vi "ECG_WD.vi"() -> ()   [LabVIEW 2020]
uses:
  <vilib>/Analysis/3filter.llb/Filter Passband Type.ctl
  <vilib>/Analysis/2dsp.llb/Real FFT.vi
  <vilib>/Utility/file.llb/Read Delimited Spreadsheet (DBL).vi
  <vilib>/Analysis/3filter.llb/Butterworth Filter (DBL).vi
  <vilib>/Analysis/NI_AALBase.lvlib
  <vilib>/Analysis/NI_AALPro.lvlib
panel:
  out "WD_stimuli 4":dbl[](graph)
  out "WD_stimuli3":dbl[](graph)
  out "WD_stimuli 2":dbl[](graph)
  out "WD_stimuli1":dbl[](graph)
  out "WD_baseline":dbl[](graph)
  out "PS_WD_stimuli4":cluster{"x":dbl, "x":dbl, dbl[]}(graph)
  out "PS_WD_stimuli 2":cluster{"x":dbl, "x":dbl, dbl[]}(graph)
  out "PS_WD_stimuli3":cluster{"x":dbl, "x":dbl, dbl[]}(graph)
  out "PS_WD_stimuli1":cluster{"x":dbl, "x":dbl, dbl[]}(graph)
  out "PS_WD_baseline 2":cluster{"x":dbl, "x":dbl, dbl[]}(graph)
  out "RRI_series_WD_stimuli4":dbl[](graph)
  out "RRI_series_WD_stimuli3":dbl[](graph)
  out "RRI_series_WD_stimuli2":dbl[](graph)
  out "RRI_series_WD_stimuli1":dbl[](graph)
  out "RRI_series_WD_baseline":dbl[](graph)
  out "WD_stimuli 4":dbl[](graph)
  out "WD_stimuli3":dbl[](graph)
  out "WD_stimuli 2":dbl[](graph)
  out "WD_stimuli1":dbl[](graph)
  out "WD_baseline":dbl[](graph)
  out "psd_size 5":i32
  out "PS_WD_stimuli4":cluster{"x":dbl, "x":dbl, dbl[]}(graph)
  out "LF/HF 5":dbl
  out "HF  2":dbl
  out "LF  2":dbl
  out "TP (<=0.4Hz)  2":dbl
  out "RRI_size 5":i32
  out "RRI_series_WD_stimuli4":dbl[](graph)
  out "RRI series 5":dbl[](array[numeric])
  out "size(s) 5":i32
  out "2nd Derivatives 5":dbl[](array[numeric])
  out "Amplitudes 5":dbl[](array[numeric])
  out "amplitude 5":dbl[](array[numeric])
  out "location 5":dbl[](array[numeric])
  out "Locations 5":dbl[](array[numeric])
  in  "file path (dialog if empty) 5":path
  out "psd_size 4":i32
  out "PS_WD_stimuli3":cluster{"x":dbl, "x":dbl, dbl[]}(graph)
  out "LF/HF 4":dbl
  out "HF  2":dbl
  out "LF  2":dbl
  out "TP (<=0.4Hz)  2":dbl
  out "RRI_size 4":i32
  out "RRI_series_WD_stimuli3":dbl[](graph)
  out "RRI series 4":dbl[](array[numeric])
  out "size(s) 4":i32
  out "2nd Derivatives 4":dbl[](array[numeric])
  out "Amplitudes 4":dbl[](array[numeric])
  out "amplitude 4":dbl[](array[numeric])
  out "location 4":dbl[](array[numeric])
  out "Locations 4":dbl[](array[numeric])
  in  "file path (dialog if empty) 4":path
  out "psd_size 3":i32
  out "PS_WD_stimuli 2":cluster{"x":dbl, "x":dbl, dbl[]}(graph)
  out "LF/HF 3":dbl
  out "HF  2":dbl
  out "LF  2":dbl
  out "TP (<=0.4Hz)  2":dbl
  out "RRI_size 3":i32
  out "RRI_series_WD_stimuli2":dbl[](graph)
  out "RRI series 3":dbl[](array[numeric])
  out "size(s) 3":i32
  out "2nd Derivatives 3":dbl[](array[numeric])
  out "Amplitudes 3":dbl[](array[numeric])
  out "amplitude 3":dbl[](array[numeric])
  out "location 3":dbl[](array[numeric])
  out "Locations 3":dbl[](array[numeric])
  in  "file path (dialog if empty) 3":path
  out "psd_size 2":i32
  out "PS_WD_stimuli1":cluster{"x":dbl, "x":dbl, dbl[]}(graph)
  out "LF/HF 2":dbl
  out "HF  2":dbl
  out "LF  2":dbl
  out "TP (<=0.4Hz)  2":dbl
  out "RRI_size 2":i32
  out "RRI_series_WD_stimuli1":dbl[](graph)
  out "RRI series 2":dbl[](array[numeric])
  out "size(s) 2":i32
  out "2nd Derivatives 2":dbl[](array[numeric])
  out "Amplitudes 2":dbl[](array[numeric])
  out "amplitude 2":dbl[](array[numeric])
  out "location 2":dbl[](array[numeric])
  out "Locations 2":dbl[](array[numeric])
  in  "file path (dialog if empty) 2":path
  out "psd_size":i32
  out "PS_WD_baseline":cluster{"x":dbl, "x":dbl, dbl[]}(graph)
  out "LF/HF":dbl
  out "HF":dbl
  out "LF":dbl
  out "TP (<=0.4Hz)":dbl
  out "RRI_size":i32
  out "RRI_series_WD_baseline":dbl[](graph)
  out "RRI series":dbl[](array[numeric])
  out "size(s)":i32
  out "2nd Derivatives":dbl[](array[numeric])
  out "Amplitudes":dbl[](array[numeric])
  out "amplitude":dbl[](array[numeric])
  out "location":dbl[](array[numeric])
  out "Locations":dbl[](array[numeric])
  in  "file path (dialog if empty)":path
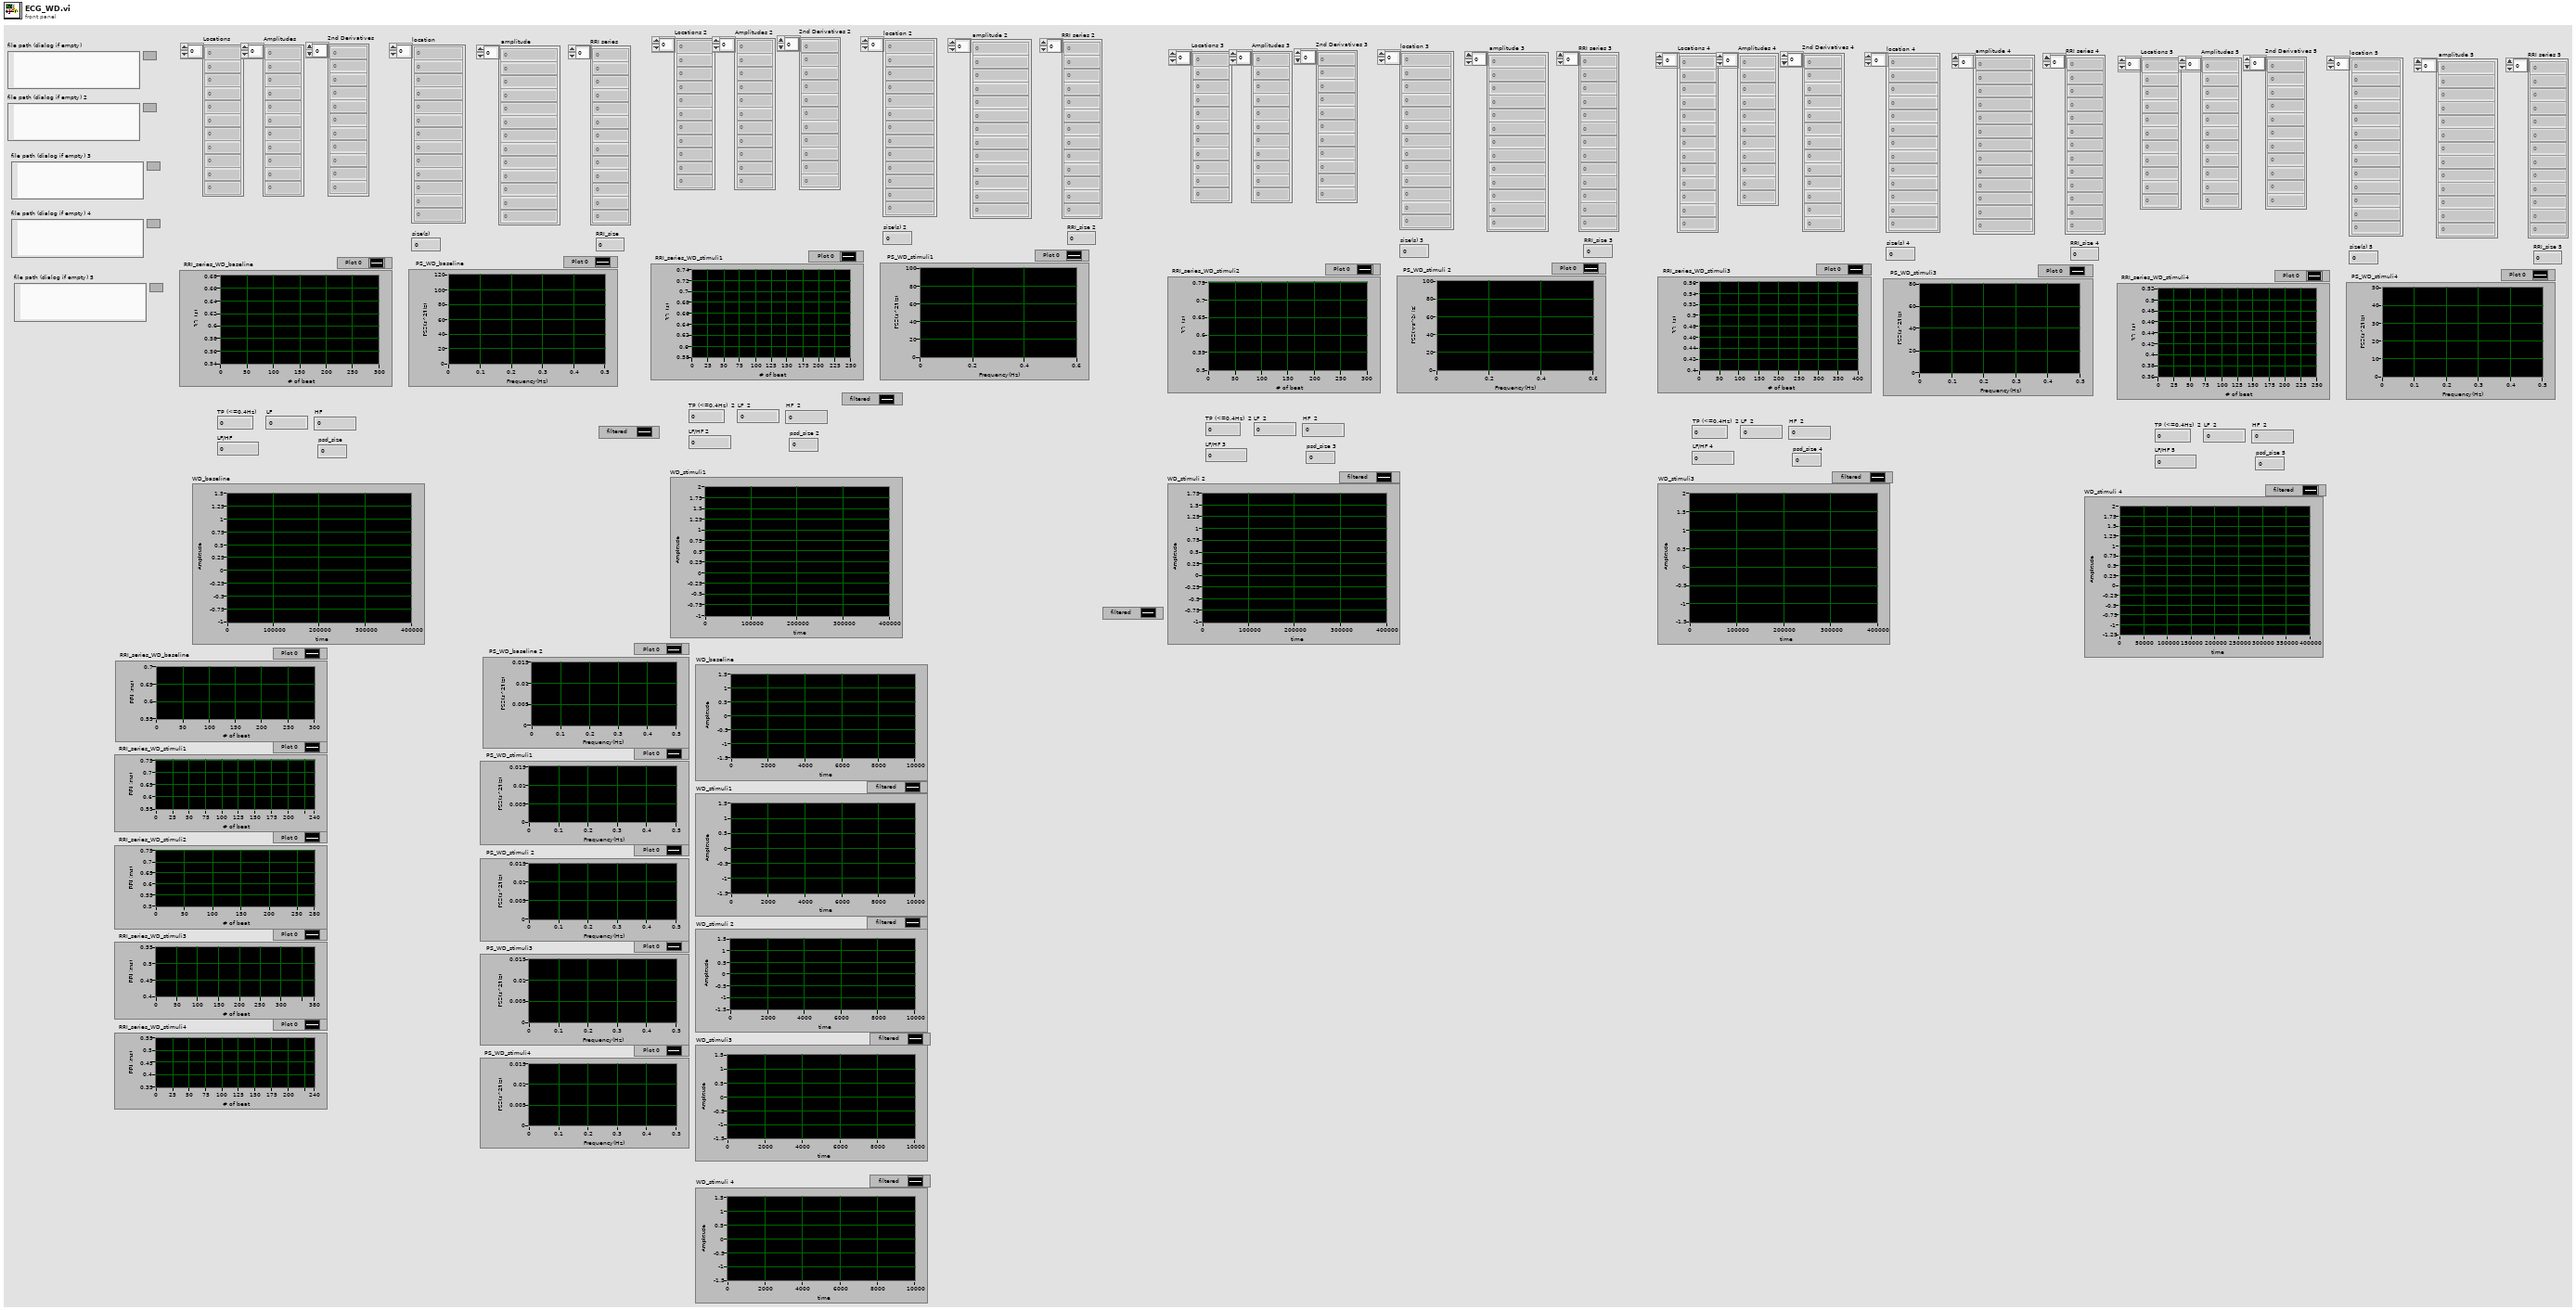
[diagram p1: front panel]
types:
  T1 = typedef "NI_AALBase.lvlib/Filter Passband Type.ctl" = enum32{"Lowpass", "Highpass", "Bandpass", "Bandstop"}
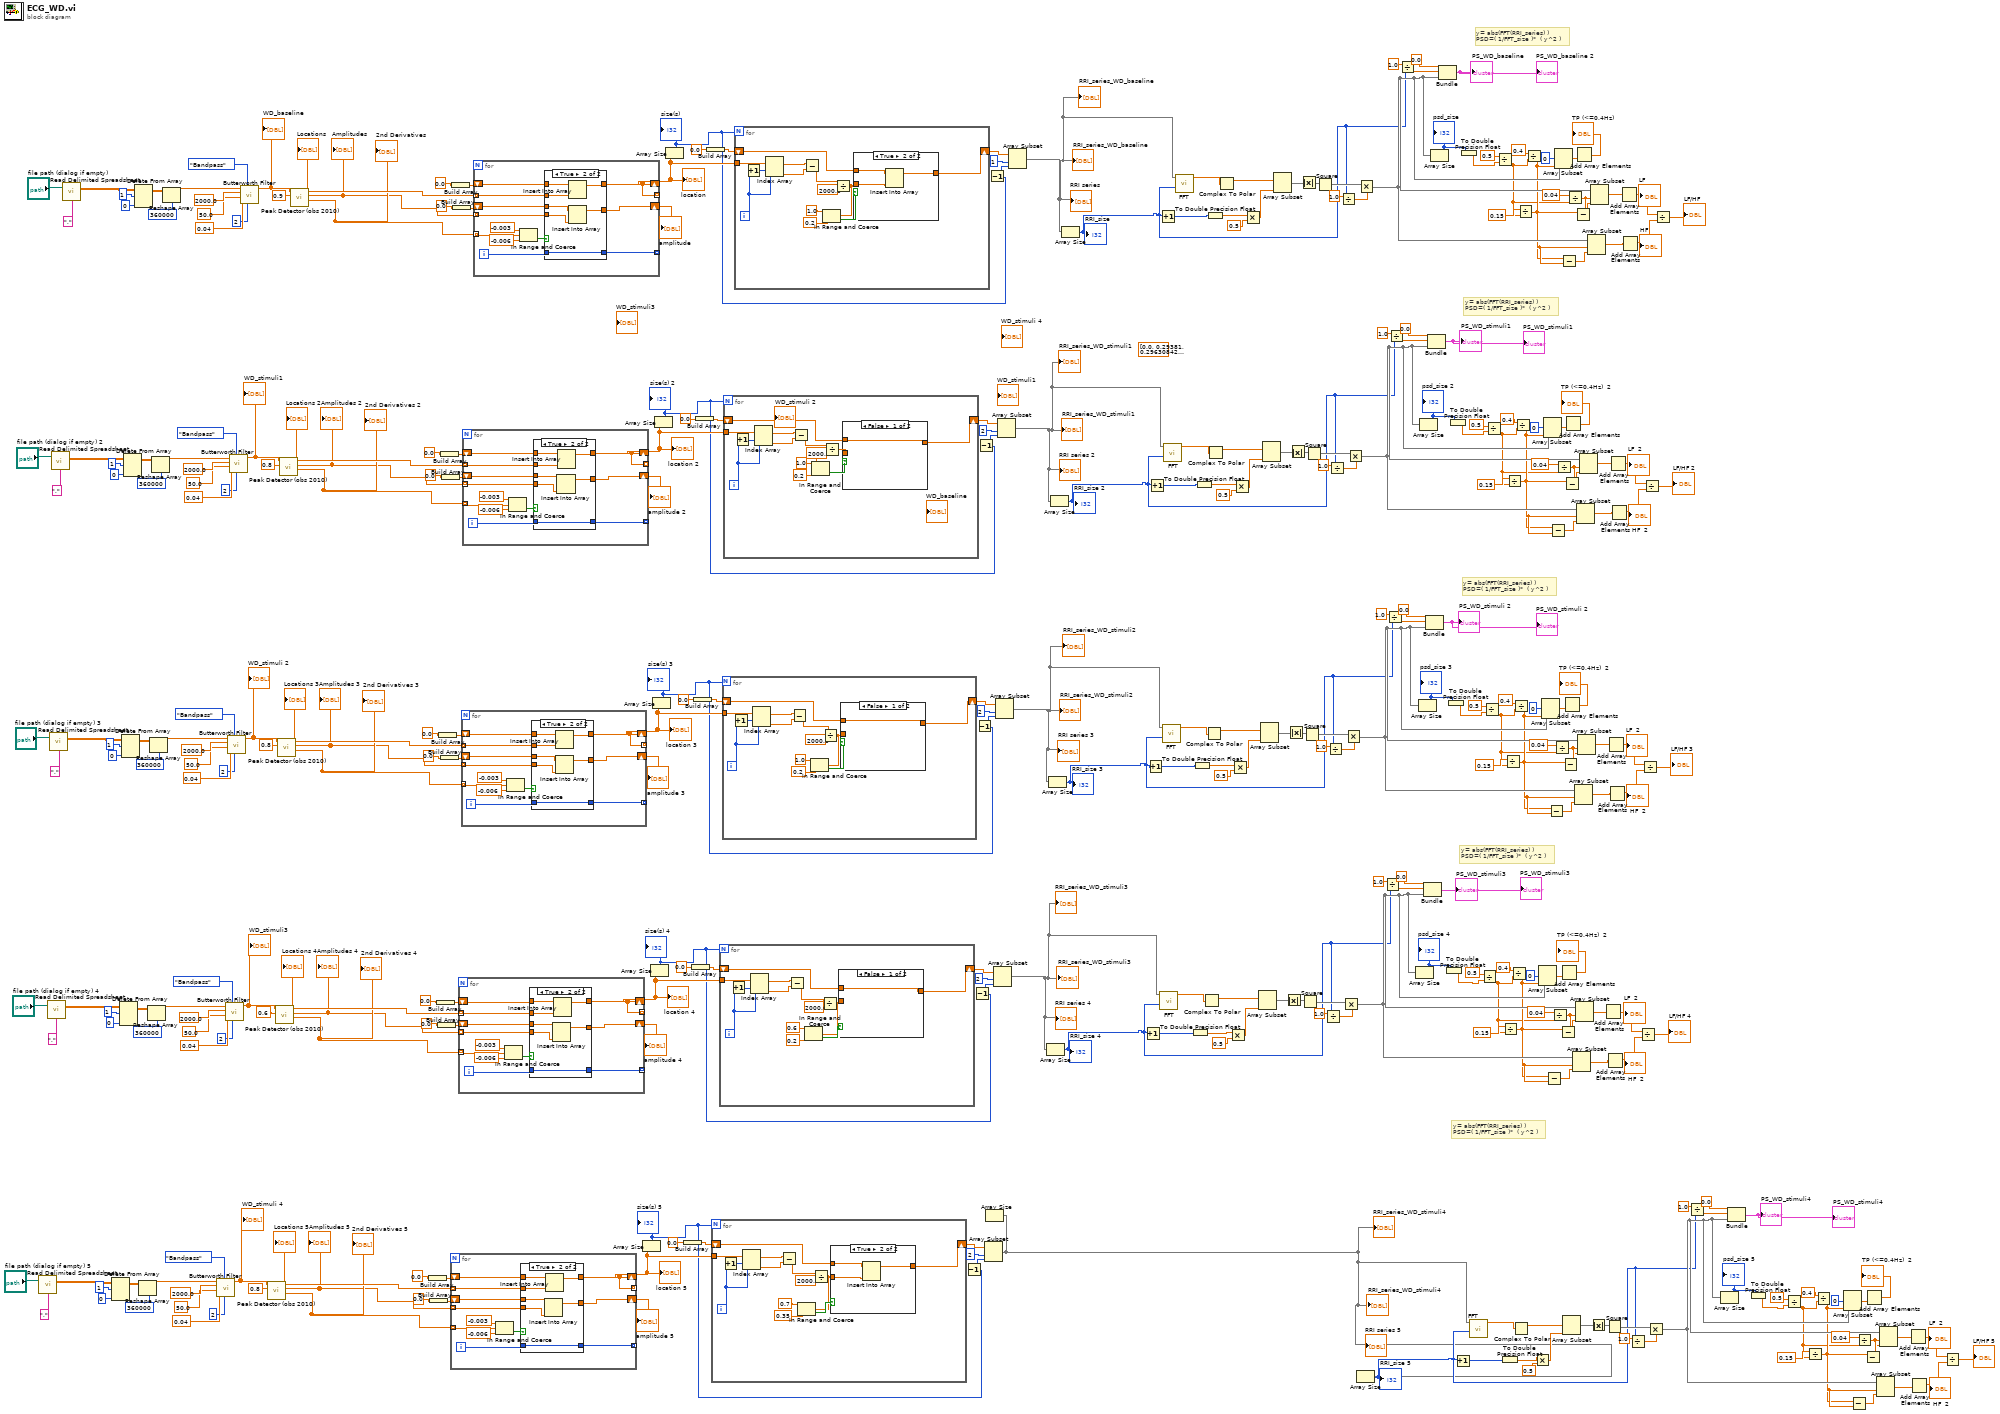
[diagram p0: block diagram]
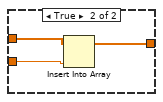
[diagram p4: hidden frame]
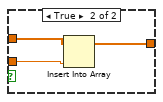
[diagram p6: hidden frame]
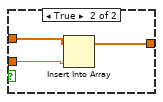
[diagram p8: hidden frame]
diagram:
  (unwired) dbl[] [0.0, 0.29381, 0.29630842105263167, 0.19107985480943712, 0.38411172413793127, 0.2005576470588235, 0.5415192546583851, 0.45620357142857126, 0.38751630434782625, 0.5665753623188401, 0.15213750000000026, 0.5900847665847664, 0.5553697788697791, 0.2967545454545455, 0.25331290322580635, 0.24809710144927521, 0.24300555555555636, 0.36543567251461884, 0.21673793859649226, 0.5703541666666663, 0.5683518808777421, 0.1222697768762675, 0.18815601023018047, 0.5246007905138335, 0.1950573913043474, 0.33014545454545363, 0.44885793103448357, 0.23535953177257518, 0.22516909814323682, 0.22548551724137944, 0.12783937499999887, 0.3413281250000004, 0.20749715909090938, 0.4030790441176464, 0.23350756302520992, 0.21006071428571715, 0.11335771889400803, 0.22295537634408547, 0.26558703703703657, 0.539833333333334, 0.10605387205387018, 0.5560011961722502, 0.2837828947368415, 0.22915000000000418, 0.47333333333332916, 0.1211837606837598, 0.4628660477453579, 0.18260098522167567, 0.46732142857142733, 0.2725865384615389, 0.13694227886056964, 0.4191120689655179, 0.306553571428573, 0.2667719780219784, 0.2580607142857154, 0.33838716216216014, 0.3010878378378372, 0.15537142857142783, 0.1092118012422354, 0.4295310559006218, 0.2176678571428603, 0.24333214285713822, 0.33524285714285895, 0.4297541666666689, 0.4027492816091929, 0.22172155172414065, 0.11575632183907913, 0.24070833333333752, 0.1274596273291948, 0.4452750000000023, 0.13352592592593027, 0.3237400000000008, 0.23238333333333827, 0.16247222222222035, 0.21347619047618593, 0.19381691297208903, 0.17932454361054795, 0.44334663865545565, 0.3988690476190584, 0.18958333333333144, 0.23410285714285095, 0.22339714285714507, 0.48038359788359486, 0.11273425925926261, 0.3386563157894713, 0.4857236842105266, 0.11062499999999886, 0.19525652173913244, 0.259178260869561, 0.35527931488800846, 0.404057239057245, 0.4889351851851842, 0.34998809523808916, 0.3202440476190489, 0.589205357142859, 0.2485571847507444, 0.23178793309438106, 0.22364814814814338, 0.24764285714285705, 0.11521008403361321, 0.22225122549019716, 0.13170789473684152, 0.24314193548387664, 0.2838542183622792, 0.4953853276353257, 0.5381438095238096, 0.23682380952381266, 0.20920119047618613, 0.3128903846153861, 0.2558694638694661, 0.20557499999999607, 0.1322803571428608, 0.28126964285713996, 0.1638875000000013, 0.20415668202765147, 0.2169942857142786, 0.263934285714285, 0.11046571428571639, 0.10588451612903071, 0.20018548387096757, 0.26614814814814736, 0.3715351851851807, 0.30481071428572193, 0.3190964285714273, 0.13439503105589523, 0.1107478260869641, 0.14819374999999724, 0.3442210648148176, 0.2693175381263586, 0.25935249554367346, 0.3362651515151498, 0.4748333333333363, 0.3614848484848494, 0.2054005681818154, 0.11299553571428333, 0.5907453917050702, 0.21269508448541075, 0.2979044540229907, 0.4190350985221656, 0.21104158215010216, 0.1368107416879809, 0.10664558629775911, 0.22124639423076076, 0.4358821339950367, 0.2326143695014764, 0.13911143695014516, 0.20822011385199346, 0.28922450980391545, 0.5867462121212128, 0.2866250000000008, 0.21224999999999739, 0.3377343750000108, 0.36128124999999045, 0.20962073863637443, 0.1334791666666746, 0.2457410714285686, 0.32503439153440183, 0.23767471590909395, 0.20249090909091194, 0.11029696969697511, 0.525561650992671, 0.3117830459770232, 0.17371920289855325, 0.23944642857141218, 0.15852950310559777, 0.188875959079283, 0.3872088235294058, 0.1356121794871683, 0.23071666666668023, 0.2992083333333255, 0.27228602150537995, 0.28636397849463435, 0.2875614942528557, 0.5852875253549712, 0.2558449197861137, 0.5800703463203405, 0.13601994851994448, 0.4267990990990995, 0.2631744031830294, 0.21025525946704704, 0.35653744239630214, 0.15822537878787557, 0.10333712121213523, 0.5940228494623483, 0.27047896213184686, 0.15288895417155857, 0.12790090090089734, 0.4482528735632201, 0.11243553223388858, 0.3093695652173949, 0.21647076461769643, 0.10553448275861399, 0.5130234482758596, 0.24094647058824137, 0.18007999999998958, 0.11140000000000327, 0.26672857142857254, 0.2067541871921179, 0.4282875116495717, 0.3605463963964013, 0.5097857142857265, 0.24231249999999704, 0.43038014101058764, 0.17514827201782168, 0.22252564102564065, 0.25950000000000273, 0.5442727272727268, 0.33003496503496876, 0.263613300492608, 0.14415852490421344, 0.2096249999999884, 0.13157142857143356, 0.14642857142857224, 0.391905594405614, 0.20831006493506266, 0.2599535714285537, 0.2499000000000109, 0.2820270270270271, 0.1985961538461538, 0.45420230769229875, 0.49392838196287414, 0.5608398366606053, 0.3559940191387625, 0.19250378787877764, 0.2012583333333282, 0.20667187499999784, 0.23565682870371063, 0.16285629629628318, 0.2627443478260858, 0.1731551116333776, 0.31491071428571615, 0.2115231092437, 0.42092857142857554, 0.1386210317460268, 0.2952741666666725, 0.2542487745098043, 0.337180392156867, 0.23917121212120662, 0.5674204545454558, 0.21861999999998716, 0.145207586206908, 0.22685991379310622, 0.22925492831541305, 0.32375874125874304, 0.43428114478113855, 0.24564953703703907, 0.1512150862069035, 0.5284409090909179, 0.40655526315788393, 0.19313045112781424, 0.5552866666666603, 0.2112126436781665, 0.4515671182266061, 0.3805942857142952, 0.46748883928570706, 0.2095468750000009, 0.40958750000000066, 0.14264637096775346, 0.25529333333332715, 0.19294000000000722, 0.13952116402117554, 0.24676934523807859, 0.18860208333333617, 0.12189177489177894, 0.2235337243401858, 0.35489285714285757, 0.3956515151514992, 0.15361785714286214, 0.15051290322578836, 0.44247043010753373, 0.5090208333333379, 0.13926250000000095, 0.2645380952380947, 0.5987088744588647, 0.4432761904761833, 0.14383053221288833, 0.4204789915966387, 0.14253571428571377, 0.31499137931034227, 0.269181697612737, 0.326163879598667, 0.5397943469785531, 0.29422685185186026, 0.3191545584045343, 0.35618218623483244, 0.24157577132484676, 0.5840832512315615, 0.16671488095235532, 0.14611147186147377, 0.2641345755693578, 0.28046066252588275, 0.4347202380952524, 0.4147321428571331, 0.12436538461540181, 0.15311538461540408, 0.2913942307692139, 0.1857916666666597, 0.35801851851852007, 0.23258267195768667, 0.10083559113297724, 0.2668965517241588, 0.31366666666664855, 0.32431981981983427, 0.24788307873089366, 0.4258425559947341, 0.27787878787879094, 0.10010645933013507, 0.18526096491228827, 0.24477083333331962, 0.18829185185185793, 0.10567904761904856, 0.17557573632538492, 0.4399065217391467, 0.5968530303030377, 0.16281696969696213, 0.4309633333333238, 0.10487982625483028, 0.22304687499999432, 0.2574791666666556, 0.11044391025640721, 0.20017692307695256, 0.15451082251084358, 0.21483001893940923, 0.30792105263157055, 0.19797478070177021, 0.11159416666663446, 0.4827461111111404, 0.2883823529411984, 0.19885999999996784, 0.16439393939390357, 0.27703774928772873, 0.2265481481481686, 0.1250083333333123, 0.2403138888888634, 0.1580396825397088, 0.1122888198757721, 0.5006397515527965, 0.10669642857143913, 0.2441284615384518, 0.20271153846152856, 0.389413043478271, 0.22863043478261602, 0.5493819444444625, 0.24320676691726817, 0.26819799498750285, 0.1169380952380834, 0.4512249084249049, 0.2749600000000214, 0.1626666666666381, 0.20178623188402867, 0.26835411899315886, 0.4641790935672532, 0.27582959326790046, 0.2572840579710487, 0.1303252252251923, 0.15375096525099252, 0.5137696428571132, 0.2957450549450584, 0.22346847290640426, 0.10255724137931566, 0.46152148148149763, 0.3519560185185071, 0.355340277777799, 0.2148028673835256, 0.17558151700083613, 0.11204617117118687, 0.306155303030323, 0.21241761363634737, 0.5250142045454425, 0.32369642857142367, 0.17801847290638761, 0.11129985007497112, 0.14849891774889556, 0.23901623376622183, 0.5667946127946379, 0.3195291666666549, 0.2099656250000237, 0.10435011574071495, 0.25229979979980044, 0.27154874517376015, 0.24066184649609568, 0.24821637931034957, 0.30346592592593424, 0.5280641666666384, 0.2209374999999909, 0.5431042780748214, 0.24045903361346177, 0.11682037815126023, 0.2894420677361893, 0.32801381461675305, 0.5127225490195997, 0.11342380952382314, 0.2214761904761815, 0.29268749999999955, 0.322488970588239, 0.1145654648956338, 0.5754108422939055, 0.24313888888889323, 0.3561922043010668, 0.180266129032276, 0.10029166666663514, 0.23215064102566885, 0.5855743589743554, 0.19788850574713024, 0.46721982758620584] ("interval 5")
  # "y= abs(FFT(RRI_series) )         \nPSD=( 1/FFT_size )*  ( y^2 )"
  # "y= abs(FFT(RRI_series) )         \nPSD=( 1/FFT_size )*  ( y^2 )"
  # "y= abs(FFT(RRI_series) )         \nPSD=( 1/FFT_size )*  ( y^2 )"
  # "y= abs(FFT(RRI_series) )         \nPSD=( 1/FFT_size )*  ( y^2 )"
  # "y= abs(FFT(RRI_series) )         \nPSD=( 1/FFT_size )*  ( y^2 )"
  n1 = call-poly <vilib>:"Read Delimited Spreadsheet.vi"("file path (dialog if empty)"="file path (dialog if empty) 5", "delimiter (\\t)"="," ("delimiter (\\t)")) -> ("all rows"=w79:dbl[][])  [unwired: 8 in, 5 out]
  n2 = call-poly <vilib>:"Read Delimited Spreadsheet.vi"("file path (dialog if empty)"="file path (dialog if empty) 4", "delimiter (\\t)"="," ("delimiter (\\t)")) -> ("all rows"=w144:dbl[][])  [unwired: 8 in, 5 out]
  n3 = call-poly <vilib>:"Read Delimited Spreadsheet.vi"("file path (dialog if empty)"="file path (dialog if empty) 3", "delimiter (\\t)"="," ("delimiter (\\t)")) -> ("all rows"=w209:dbl[][])  [unwired: 8 in, 5 out]
  n4 = call-poly <vilib>:"Read Delimited Spreadsheet.vi"("file path (dialog if empty)"="file path (dialog if empty) 2", "delimiter (\\t)"="," ("delimiter (\\t)")) -> ("all rows"=w274:dbl[][])  [unwired: 8 in, 5 out]
  n5 = call-poly <vilib>:"Read Delimited Spreadsheet.vi"("file path (dialog if empty)"="file path (dialog if empty)", "delimiter (\\t)"="," ("delimiter (\\t)")) -> ("all rows"=w339:dbl[][])  [unwired: 8 in, 5 out]
  n6 = Delete From Array(array=w79, length=1, index (col)=0 ("disabled index (col)")) -> (array with subset deleted=w69:dbl[][])  [unwired: 1 in, 1 out]
  n7 = Delete From Array(array=w144, length=1, index (col)=0 ("disabled index (col)")) -> (array with subset deleted=w134:dbl[][])  [unwired: 1 in, 1 out]
  n8 = Delete From Array(array=w209, length=1, index (col)=0 ("disabled index (col)")) -> (array with subset deleted=w199:dbl[][])  [unwired: 1 in, 1 out]
  n9 = Delete From Array(array=w274, length=1, index (col)=0 ("disabled index (col)")) -> (array with subset deleted=w264:dbl[][])  [unwired: 1 in, 1 out]
  n10 = Delete From Array(array=w339, length=1, index (col)=0 ("disabled index (col)")) -> (array with subset deleted=w329:dbl[][])  [unwired: 1 in, 1 out]
  n11 = Reshape Array(w69, 360000 ("dimension size")) -> (w68:dbl[])
  n12 = Reshape Array(w134, 360000 ("dimension size")) -> (w133:dbl[])
  n13 = Reshape Array(w199, 360000 ("dimension size")) -> (w198:dbl[])
  n14 = Reshape Array(w264, 360000 ("dimension size")) -> (w263:dbl[])
  n15 = Reshape Array(w329, 360000 ("dimension size")) -> (w328:dbl[])
  n16 = call-poly <vilib>:"Butterworth Filter.vi"("order"=2, "filter type"=Filter_Passband_Type."Bandpass", "low cutoff freq: fl"=0.04, "high cutoff freq: fh"=50.0, "sampling freq: fs"=2000.0, "X"=w68) -> ("Filtered X"=w12:dbl[])  [unwired: 2 in, 1 out]
  "WD_stimuli 4" <- w12
  n17 = call-poly <vilib>:"Butterworth Filter.vi"("order"=2, "filter type"=Filter_Passband_Type."Bandpass", "low cutoff freq: fl"=0.04, "high cutoff freq: fh"=50.0, "sampling freq: fs"=2000.0, "X"=w133) -> ("Filtered X"=w13:dbl[])  [unwired: 2 in, 1 out]
  "WD_stimuli3" <- w13
  n18 = call-poly <vilib>:"Butterworth Filter.vi"("order"=2, "filter type"=Filter_Passband_Type."Bandpass", "low cutoff freq: fl"=0.04, "high cutoff freq: fh"=50.0, "sampling freq: fs"=2000.0, "X"=w198) -> ("Filtered X"=w14:dbl[])  [unwired: 2 in, 1 out]
  "WD_stimuli 2" <- w14
  n19 = call-poly <vilib>:"Butterworth Filter.vi"("order"=2, "filter type"=Filter_Passband_Type."Bandpass", "low cutoff freq: fl"=0.04, "high cutoff freq: fh"=50.0, "sampling freq: fs"=2000.0, "X"=w263) -> ("Filtered X"=w15:dbl[])  [unwired: 2 in, 1 out]
  "WD_stimuli1" <- w15
  n20 = call-poly <vilib>:"Butterworth Filter.vi"("order"=2, "filter type"=Filter_Passband_Type."Bandpass", "low cutoff freq: fl"=0.04, "high cutoff freq: fh"=50.0, "sampling freq: fs"=2000.0, "X"=w328) -> ("Filtered X"=w16:dbl[])  [unwired: 2 in, 1 out]
  "WD_baseline" <- w16
  n21 = call <vilib>:"Peak Detector (obs 2010).vi"("threshold"=0.8, "X"=w12) -> ("2nd Derivatives"=w62:dbl[], "Amplitudes"=w59:dbl[], "Locations"=w64:dbl[])  [unwired: 5 in, 2 out]
  "Locations 5" <- w64
  "Amplitudes 5" <- w59
  "2nd Derivatives 5" <- w62
  n22 = call <vilib>:"Peak Detector (obs 2010).vi"("threshold"=0.6, "X"=w13) -> ("2nd Derivatives"=w127:dbl[], "Amplitudes"=w124:dbl[], "Locations"=w129:dbl[])  [unwired: 5 in, 2 out]
  "Locations 4" <- w129
  "Amplitudes 4" <- w124
  "2nd Derivatives 4" <- w127
  n23 = call <vilib>:"Peak Detector (obs 2010).vi"("threshold"=0.8, "X"=w14) -> ("2nd Derivatives"=w192:dbl[], "Amplitudes"=w189:dbl[], "Locations"=w194:dbl[])  [unwired: 5 in, 2 out]
  "Locations 3" <- w194
  "Amplitudes 3" <- w189
  "2nd Derivatives 3" <- w192
  n24 = call <vilib>:"Peak Detector (obs 2010).vi"("threshold"=0.8, "X"=w15) -> ("2nd Derivatives"=w257:dbl[], "Amplitudes"=w254:dbl[], "Locations"=w259:dbl[])  [unwired: 5 in, 2 out]
  "Locations 2" <- w259
  "Amplitudes 2" <- w254
  "2nd Derivatives 2" <- w257
  n25 = call <vilib>:"Peak Detector (obs 2010).vi"("threshold"=0.9, "X"=w16) -> ("2nd Derivatives"=w322:dbl[], "Amplitudes"=w319:dbl[], "Locations"=w324:dbl[])  [unwired: 5 in, 2 out]
  "Locations" <- w324
  "Amplitudes" <- w319
  "2nd Derivatives" <- w322
  n26 = Build Array(0.0 ("element")) -> (w66:dbl[])
  n27 = Build Array(0.0 ("element")) -> (w60:dbl[])
  n28 = Build Array(0.0 ("element")) -> (w131:dbl[])
  n29 = Build Array(0.0 ("element")) -> (w125:dbl[])
  n30 = Build Array(0.0 ("element")) -> (w196:dbl[])
  n31 = Build Array(0.0 ("element")) -> (w190:dbl[])
  n32 = Build Array(0.0 ("element")) -> (w261:dbl[])
  n33 = Build Array(0.0 ("element")) -> (w255:dbl[])
  n34 = for {
    tunnel: w62 -> [w346] mode=indexing
    shift-right: [w341] -> w58
    shift-left: w66 -> [w349]
    tunnel: [w347] -> _ mode=indexing
    tunnel: w64 -> [w345] mode=indexing
    shift-right: [w343] -> w63
    shift-left: w60 -> [w344]
    tunnel: w59 -> [w342] mode=indexing
    tunnel: [w341] -> _ mode=indexing
    i -> [w348]
    n35 = In Range and Coerce(upper limit=-0.003, x=w346, lower limit=-0.006) -> (In Range?=w350:bool)  [unwired: 1 out]
    n36 = case shown="True" w350 {
      tunnel: w349 -> [w355 w362]
      tunnel: [w355 w361] -> w341
      tunnel: [w354 w360] -> w347
      tunnel: w348 -> [w354 w360]
      tunnel: w345 -> [_ w359]
      tunnel: w344 -> [w353 w358]
      tunnel: [w353 w357] -> w343
      tunnel: w342 -> [_ w356]
      frame False {
      }
      frame True {
        n37 = Insert Into Array(array=w358, new element=w356) -> (w357:dbl[])  [unwired: 1 in]
        n38 = Insert Into Array(array=w362, new element=w359) -> (w361:dbl[])  [unwired: 1 in]
      }
    }
  }
  "location 5" <- w58
  "amplitude 5" <- w63
  n39 = Build Array(0.0 ("element")) -> (w326:dbl[])
  n40 = Build Array(0.0 ("element")) -> (w320:dbl[])
  n41 = for {
    tunnel: w127 -> [w368] mode=indexing
    shift-right: [w363] -> w123
    shift-left: w131 -> [w371]
    tunnel: [w369] -> _ mode=indexing
    tunnel: w129 -> [w367] mode=indexing
    shift-right: [w365] -> w128
    shift-left: w125 -> [w366]
    tunnel: w124 -> [w364] mode=indexing
    tunnel: [w363] -> _ mode=indexing
    i -> [w370]
    n42 = In Range and Coerce(upper limit=-0.003, x=w368, lower limit=-0.006) -> (In Range?=w372:bool)  [unwired: 1 out]
    n43 = case shown="True" w372 {
      tunnel: w371 -> [w377 w384]
      tunnel: [w377 w383] -> w363
      tunnel: [w376 w382] -> w369
      tunnel: w370 -> [w376 w382]
      tunnel: w367 -> [_ w381]
      tunnel: w366 -> [w375 w380]
      tunnel: [w375 w379] -> w365
      tunnel: w364 -> [_ w378]
      frame False {
      }
      frame True {
        n44 = Insert Into Array(array=w380, new element=w378) -> (w379:dbl[])  [unwired: 1 in]
        n45 = Insert Into Array(array=w384, new element=w381) -> (w383:dbl[])  [unwired: 1 in]
      }
    }
  }
  "location 4" <- w123
  "amplitude 4" <- w128
  n46 = for {
    tunnel: w192 -> [w390] mode=indexing
    shift-right: [w385] -> w188
    shift-left: w196 -> [w393]
    tunnel: [w391] -> _ mode=indexing
    tunnel: w194 -> [w389] mode=indexing
    shift-right: [w387] -> w193
    shift-left: w190 -> [w388]
    tunnel: w189 -> [w386] mode=indexing
    tunnel: [w385] -> _ mode=indexing
    i -> [w392]
    n47 = In Range and Coerce(upper limit=-0.003, x=w390, lower limit=-0.006) -> (In Range?=w394:bool)  [unwired: 1 out]
    n48 = case shown="True" w394 {
      tunnel: w393 -> [w399 w406]
      tunnel: [w399 w405] -> w385
      tunnel: [w398 w404] -> w391
      tunnel: w392 -> [w398 w404]
      tunnel: w389 -> [_ w403]
      tunnel: w388 -> [w397 w402]
      tunnel: [w397 w401] -> w387
      tunnel: w386 -> [_ w400]
      frame False {
      }
      frame True {
        n49 = Insert Into Array(array=w402, new element=w400) -> (w401:dbl[])  [unwired: 1 in]
        n50 = Insert Into Array(array=w406, new element=w403) -> (w405:dbl[])  [unwired: 1 in]
      }
    }
  }
  "location 3" <- w188
  "amplitude 3" <- w193
  n51 = for {
    tunnel: w257 -> [w412] mode=indexing
    shift-right: [w407] -> w253
    shift-left: w261 -> [w415]
    tunnel: [w413] -> _ mode=indexing
    tunnel: w259 -> [w411] mode=indexing
    shift-right: [w409] -> w258
    shift-left: w255 -> [w410]
    tunnel: w254 -> [w408] mode=indexing
    tunnel: [w407] -> _ mode=indexing
    i -> [w414]
    n52 = In Range and Coerce(upper limit=-0.003, x=w412, lower limit=-0.006) -> (In Range?=w416:bool)  [unwired: 1 out]
    n53 = case shown="True" w416 {
      tunnel: w415 -> [w421 w428]
      tunnel: [w421 w427] -> w407
      tunnel: [w420 w426] -> w413
      tunnel: w414 -> [w420 w426]
      tunnel: w411 -> [_ w425]
      tunnel: w410 -> [w419 w424]
      tunnel: [w419 w423] -> w409
      tunnel: w408 -> [_ w422]
      frame False {
      }
      frame True {
        n54 = Insert Into Array(array=w424, new element=w422) -> (w423:dbl[])  [unwired: 1 in]
        n55 = Insert Into Array(array=w428, new element=w425) -> (w427:dbl[])  [unwired: 1 in]
      }
    }
  }
  "location 2" <- w253
  "amplitude 2" <- w258
  n56 = for {
    tunnel: w322 -> [w434] mode=indexing
    shift-right: [w429] -> w318
    shift-left: w326 -> [w437]
    tunnel: [w435] -> _ mode=indexing
    tunnel: w324 -> [w433] mode=indexing
    shift-right: [w431] -> w323
    shift-left: w320 -> [w432]
    tunnel: w319 -> [w430] mode=indexing
    tunnel: [w429] -> _ mode=indexing
    i -> [w436]
    n57 = In Range and Coerce(upper limit=-0.003, x=w434, lower limit=-0.006) -> (In Range?=w438:bool)  [unwired: 1 out]
    n58 = case shown="True" w438 {
      tunnel: w437 -> [w443 w450]
      tunnel: [w443 w449] -> w429
      tunnel: [w442 w448] -> w435
      tunnel: w436 -> [w442 w448]
      tunnel: w433 -> [_ w447]
      tunnel: w432 -> [w441 w446]
      tunnel: [w441 w445] -> w431
      tunnel: w430 -> [_ w444]
      frame False {
      }
      frame True {
        n59 = Insert Into Array(array=w446, new element=w444) -> (w445:dbl[])  [unwired: 1 in]
        n60 = Insert Into Array(array=w450, new element=w447) -> (w449:dbl[])  [unwired: 1 in]
      }
    }
  }
  "location" <- w318
  "amplitude" <- w323
  n61 = Array Size(array=w58) -> (size(s)=w54:i32)
  "size(s) 5" <- w54
  n62 = Array Size(array=w123) -> (size(s)=w118:i32)
  "size(s) 4" <- w118
  n63 = Array Size(array=w188) -> (size(s)=w183:i32)
  "size(s) 3" <- w183
  n64 = Array Size(array=w253) -> (size(s)=w248:i32)
  "size(s) 2" <- w248
  n65 = Array Size(array=w318) -> (size(s)=w313:i32)
  "size(s)" <- w313
  n66 = Build Array(0.0 ("array")) -> (w56:dbl[])
  n67 = Build Array(0.0 ("array")) -> (w121:dbl[])
  n68 = Build Array(0.0 ("array")) -> (w186:dbl[])
  n69 = Build Array(0.0 ("array")) -> (w251:dbl[])
  n70 = Build Array(0.0 ("array")) -> (w316:dbl[])
  n71 = for {
    N: w54 -> [_]
    tunnel: w58 -> [w460]
    shift-right: [w455] -> w3
    shift-left: w56 -> [w456]
    i -> [w462]
    n72 = Increment(x=w462) -> (x+1=w463:i32)
    n73 = Index Array(array=w460, index #1=w463, index #2=w462) -> (element #1=w461:dbl, element #2=w459:dbl)
    n74 = Subtract(x=w461, y=w459) -> (x-y=w452:dbl)
    n75 = Divide(x=w452, y=2000.0) -> (x/y=w451:dbl)
    n76 = In Range and Coerce(upper limit=0.7, x=w451, lower limit=0.35) -> (In Range?=w454:bool)  [unwired: 1 out]
    n77 = case shown="True" w454 {
      tunnel: w456 -> [w464 w467]
      tunnel: w451 -> [_ w466]
      tunnel: [w464 w465] -> w455
      frame False {
      }
      frame True {
        n78 = Insert Into Array(array=w467, new element=w466) -> (w465:dbl[])  [unwired: 1 in]
      }
    }
  }
  n79 = for {
    N: w118 -> [_]
    tunnel: w123 -> [w477]
    shift-right: [w471] -> w120
    shift-left: w121 -> [w472]
    i -> [w479]
    n80 = Increment(x=w479) -> (x+1=w480:i32)
    n81 = Index Array(array=w477, index #1=w480, index #2=w479) -> (element #1=w478:dbl, element #2=w476:dbl)
    n82 = Subtract(x=w478, y=w476) -> (x-y=w469:dbl)
    n83 = Divide(x=w469, y=2000.0) -> (x/y=w468:dbl)
    n84 = In Range and Coerce(upper limit=0.6, x=w468, lower limit=0.2) -> (In Range?=w473:bool)  [unwired: 1 out]
    n85 = case shown="False" w473 {
      tunnel: w472 -> [w481 w484]
      tunnel: w468 -> [_ w483]
      tunnel: [w481 w482] -> w471
      frame False {
      }
      frame True {
        n86 = Insert Into Array(array=w484, new element=w483) -> (w482:dbl[])  [unwired: 1 in]
      }
    }
  }
  n87 = for {
    N: w183 -> [_]
    tunnel: w188 -> [w494]
    shift-right: [w488] -> w185
    shift-left: w186 -> [w489]
    i -> [w496]
    n88 = Increment(x=w496) -> (x+1=w497:i32)
    n89 = Index Array(array=w494, index #1=w497, index #2=w496) -> (element #1=w495:dbl, element #2=w493:dbl)
    n90 = Subtract(x=w495, y=w493) -> (x-y=w486:dbl)
    n91 = Divide(x=w486, y=2000.0) -> (x/y=w485:dbl)
    n92 = In Range and Coerce(upper limit=1.0, x=w485, lower limit=0.2) -> (In Range?=w490:bool)  [unwired: 1 out]
    n93 = case shown="False" w490 {
      tunnel: w489 -> [w498 w501]
      tunnel: w485 -> [_ w500]
      tunnel: [w498 w499] -> w488
      frame False {
      }
      frame True {
        n94 = Insert Into Array(array=w501, new element=w500) -> (w499:dbl[])  [unwired: 1 in]
      }
    }
  }
  n95 = for {
    N: w248 -> [_]
    tunnel: w253 -> [w511]
    shift-right: [w505] -> w250
    shift-left: w251 -> [w506]
    i -> [w513]
    n96 = Increment(x=w513) -> (x+1=w514:i32)
    n97 = Index Array(array=w511, index #1=w514, index #2=w513) -> (element #1=w512:dbl, element #2=w510:dbl)
    n98 = Subtract(x=w512, y=w510) -> (x-y=w503:dbl)
    n99 = Divide(x=w503, y=2000.0) -> (x/y=w502:dbl)
    n100 = In Range and Coerce(upper limit=1.0, x=w502, lower limit=0.2) -> (In Range?=w507:bool)  [unwired: 1 out]
    n101 = case shown="False" w507 {
      tunnel: w506 -> [w515 w518]
      tunnel: w502 -> [_ w517]
      tunnel: [w515 w516] -> w505
      frame False {
      }
      frame True {
        n102 = Insert Into Array(array=w518, new element=w517) -> (w516:dbl[])  [unwired: 1 in]
      }
    }
  }
  n103 = for {
    N: w313 -> [_]
    tunnel: w318 -> [w528]
    shift-right: [w522] -> w315
    shift-left: w316 -> [w523]
    i -> [w530]
    n104 = Increment(x=w530) -> (x+1=w531:i32)
    n105 = Index Array(array=w528, index #1=w531, index #2=w530) -> (element #1=w529:dbl, element #2=w527:dbl)
    n106 = Subtract(x=w529, y=w527) -> (x-y=w521:dbl)
    n107 = Divide(x=w521, y=2000.0) -> (x/y=w519:dbl)
    n108 = In Range and Coerce(upper limit=1.0, x=w519, lower limit=0.2) -> (In Range?=w524:bool)  [unwired: 1 out]
    n109 = case shown="True" w524 {
      tunnel: w523 -> [w532 w535]
      tunnel: w519 -> [_ w534]
      tunnel: [w532 w533] -> w522
      frame False {
      }
      frame True {
        n110 = Insert Into Array(array=w535, new element=w534) -> (w533:dbl[])  [unwired: 1 in]
      }
    }
  }
  n111 = Decrement(x=w54) -> (x-1=w53:i32)
  n112 = Decrement(x=w118) -> (x-1=w117:i32)
  n113 = Decrement(x=w183) -> (x-1=w182:i32)
  n114 = Decrement(x=w248) -> (x-1=w247:i32)
  n115 = Array Subset(array=w3, index=2, length=w53) -> (w1:dbl[])
  "RRI series 5" <- w1
  "RRI_series_WD_stimuli4" <- w1
  "RRI_series_WD_stimuli4" <- w1
  n116 = Array Size(array=w1) -> ()  [unwired: 1 out]
  n117 = Decrement(x=w313) -> (x-1=w312:i32)
  n118 = Array Subset(array=w120, index=2, length=w117) -> (w9:dbl[])
  "RRI series 4" <- w9
  "RRI_series_WD_stimuli3" <- w9
  "RRI_series_WD_stimuli3" <- w9
  n119 = Array Subset(array=w185, index=2, length=w182) -> (w10:dbl[])
  "RRI series 3" <- w10
  "RRI_series_WD_stimuli2" <- w10
  "RRI_series_WD_stimuli2" <- w10
  n120 = Array Subset(array=w250, index=2, length=w247) -> (w11:dbl[])
  "RRI series 2" <- w11
  "RRI_series_WD_stimuli1" <- w11
  "RRI_series_WD_stimuli1" <- w11
  n121 = Array Subset(array=w315, index=1, length=w312) -> (w2:dbl[])
  "RRI series" <- w2
  "RRI_series_WD_baseline" <- w2
  "RRI_series_WD_baseline" <- w2
  n122 = Array Size(array=w9) -> (size(s)=w97:i32)
  "RRI_size 4" <- w97
  n123 = Array Size(array=w10) -> (size(s)=w162:i32)
  "RRI_size 3" <- w162
  n124 = Array Size(array=w11) -> (size(s)=w227:i32)
  "RRI_size 2" <- w227
  n125 = Array Size(array=w2) -> (size(s)=w292:i32)
  "RRI_size" <- w292
  n126 = Increment(x=w97) -> (x+1=w116:i32)
  n127 = Increment(x=w162) -> (x+1=w181:i32)
  n128 = Increment(x=w227) -> (x+1=w246:i32)
  n129 = Increment(x=w292) -> (x+1=w311:i32)
  n130 = call-poly <vilib>:"FFT.vi"("FFT size"=w97, "X"=w9) -> ("FFT {X}"=w96:cdb[])  [unwired: 8 in, 1 out]
  n131 = call-poly <vilib>:"FFT.vi"("FFT size"=w162, "X"=w10) -> ("FFT {X}"=w161:cdb[])  [unwired: 8 in, 1 out]
  n132 = call-poly <vilib>:"FFT.vi"("FFT size"=w227, "X"=w11) -> ("FFT {X}"=w226:cdb[])  [unwired: 8 in, 1 out]
  n133 = call-poly <vilib>:"FFT.vi"("FFT size"=w292, "X"=w2) -> ("FFT {X}"=w291:cdb[])  [unwired: 8 in, 1 out]
  n134 = To Double Precision Float(number=w116) -> (double precision float=w112:dbl)
  n135 = To Double Precision Float(number=w181) -> (double precision float=w177:dbl)
  n136 = To Double Precision Float(number=w246) -> (double precision float=w242:dbl)
  n137 = Complex To Polar(r * e^(i*theta)=w96) -> (r=w111:dbl[])  [unwired: 1 out]
  n138 = Complex To Polar(r * e^(i*theta)=w161) -> (r=w176:dbl[])  [unwired: 1 out]
  n139 = To Double Precision Float(number=w311) -> (double precision float=w307:dbl)
  n140 = Complex To Polar(r * e^(i*theta)=w226) -> (r=w241:dbl[])  [unwired: 1 out]
  n141 = Complex To Polar(r * e^(i*theta)=w291) -> (r=w306:dbl[])  [unwired: 1 out]
  n142 = Multiply(x=w112, y=0.5) -> (x*y=w114:dbl)
  n143 = Multiply(x=w177, y=0.5) -> (x*y=w179:dbl)
  n144 = Multiply(x=w242, y=0.5) -> (x*y=w244:dbl)
  n145 = Multiply(x=w307, y=0.5) -> (x*y=w309:dbl)
  n146 = Array Subset(array=w111, length=w114) -> (w102:dbl[])  [unwired: 1 in]
  n147 = Array Subset(array=w176, length=w179) -> (w167:dbl[])  [unwired: 1 in]
  n148 = Array Subset(array=w241, length=w244) -> (w232:dbl[])  [unwired: 1 in]
  n149 = Array Subset(array=w306, length=w309) -> (w297:dbl[])  [unwired: 1 in]
  n150 = Absolute Value(x=w102) -> (abs(x)=w101:dbl[])
  n151 = Absolute Value(x=w167) -> (abs(x)=w166:dbl[])
  n152 = Absolute Value(x=w232) -> (abs(x)=w231:dbl[])
  n153 = Absolute Value(x=w297) -> (abs(x)=w296:dbl[])
  n154 = Square(x=w101) -> (x^2=w100:dbl[])
  n155 = Square(x=w166) -> (x^2=w165:dbl[])
  n156 = Square(x=w231) -> (x^2=w230:dbl[])
  n157 = Square(x=w296) -> (x^2=w295:dbl[])
  n158 = Divide(x=1.0, y=w97) -> (x/y=w99:dbl)
  n159 = Divide(x=1.0, y=w162) -> (x/y=w164:dbl)
  n160 = Divide(x=1.0, y=w227) -> (x/y=w229:dbl)
  n161 = Divide(x=1.0, y=w292) -> (x/y=w294:dbl)
  n162 = Multiply(x=w100, y=w99) -> (x*y=w98:dbl[])
  n163 = Multiply(x=w165, y=w164) -> (x*y=w163:dbl[])
  n164 = Multiply(x=w230, y=w229) -> (x*y=w228:dbl[])
  n165 = Array Size(array=w1) -> (size(s)=w33:i32)
  "RRI_size 5" <- w33
  n166 = Multiply(x=w295, y=w294) -> (x*y=w293:dbl[])
  n167 = Divide(x=1.0, y=w97) -> (x/y=w103:dbl)
  n168 = Divide(x=1.0, y=w162) -> (x/y=w168:dbl)
  n169 = Divide(x=1.0, y=w227) -> (x/y=w233:dbl)
  n170 = Divide(x=1.0, y=w292) -> (x/y=w298:dbl)
  n171 = Array Size(array=w98) -> (size(s)=w95:i32)
  "psd_size 4" <- w95
  n172 = Array Size(array=w163) -> (size(s)=w160:i32)
  "psd_size 3" <- w160
  n173 = Array Size(array=w228) -> (size(s)=w225:i32)
  "psd_size 2" <- w225
  n174 = Bundle("x"=0.0, w103, w98) -> (→"PS_WD_stimuli3" →"PS_WD_stimuli3":cluster{"x":dbl, dbl, dbl[]})  [unwired: 1 in]
  n175 = Bundle("x"=0.0, w168, w163) -> (→"PS_WD_stimuli 2" →"PS_WD_stimuli 2":cluster{"x":dbl, dbl, dbl[]})  [unwired: 1 in]
  n176 = Bundle("x"=0.0, w233, w228) -> (→"PS_WD_stimuli1" →"PS_WD_stimuli1":cluster{"x":dbl, dbl, dbl[]})  [unwired: 1 in]
  n177 = Array Size(array=w293) -> (size(s)=w290:i32)
  "psd_size" <- w290
  n178 = Bundle("x"=0.0, w298, w293) -> (→"PS_WD_baseline" →"PS_WD_baseline 2":cluster{"x":dbl, dbl, dbl[]})  [unwired: 1 in]
  n179 = To Double Precision Float(number=w95) -> (double precision float=w84:dbl)
  n180 = To Double Precision Float(number=w160) -> (double precision float=w149:dbl)
  n181 = To Double Precision Float(number=w225) -> (double precision float=w214:dbl)
  n182 = Increment(x=w33) -> (x+1=w52:i32)
  n183 = To Double Precision Float(number=w290) -> (double precision float=w279:dbl)
  n184 = call-poly <vilib>:"FFT.vi"("FFT size"=w33, "X"=w1) -> ("FFT {X}"=w32:cdb[])  [unwired: 8 in, 1 out]
  n185 = Divide(x=0.5, y=w84) -> (x/y=w82:dbl)
  n186 = Divide(x=0.5, y=w149) -> (x/y=w147:dbl)
  n187 = Divide(x=0.5, y=w214) -> (x/y=w212:dbl)
  n188 = Divide(x=0.5, y=w279) -> (x/y=w277:dbl)
  n189 = To Double Precision Float(number=w52) -> (double precision float=w48:dbl)
  n190 = Divide(x=0.15, y=w82) -> (x/y=w88:dbl)
  n191 = Divide(x=0.15, y=w147) -> (x/y=w153:dbl)
  n192 = Divide(x=0.15, y=w212) -> (x/y=w218:dbl)
  n193 = Divide(x=0.4, y=w82) -> (x/y=w85:dbl)
  n194 = Divide(x=0.4, y=w147) -> (x/y=w150:dbl)
  n195 = Complex To Polar(r * e^(i*theta)=w32) -> (r=w47:dbl[])  [unwired: 1 out]
  n196 = Divide(x=0.4, y=w212) -> (x/y=w215:dbl)
  n197 = Divide(x=0.15, y=w277) -> (x/y=w283:dbl)
  n198 = Divide(x=0.4, y=w277) -> (x/y=w280:dbl)
  n199 = Multiply(x=w48, y=0.5) -> (x*y=w50:dbl)
  n200 = Array Subset(array=w98, index=0, length=w85) -> (w110:dbl[])
  n201 = Array Subset(array=w163, index=0, length=w150) -> (w175:dbl[])
  n202 = Array Subset(array=w228, index=0, length=w215) -> (w240:dbl[])
  n203 = Subtract(x=w85, y=w88) -> (x-y=w89:dbl)
  n204 = Subtract(x=w150, y=w153) -> (x-y=w154:dbl)
  n205 = Subtract(x=w215, y=w218) -> (x-y=w219:dbl)
  n206 = Divide(x=0.04, y=w82) -> (x/y=w91:dbl)
  n207 = Divide(x=0.04, y=w147) -> (x/y=w156:dbl)
  n208 = Array Subset(array=w293, index=0, length=w280) -> (w305:dbl[])
  n209 = Divide(x=0.04, y=w212) -> (x/y=w221:dbl)
  n210 = Subtract(x=w88, y=w91) -> (x-y=w90:dbl)
  n211 = Subtract(x=w280, y=w283) -> (x-y=w284:dbl)
  n212 = Add Array Elements(numeric array=w110) -> (sum=→"TP (<=0.4Hz)  2":dbl)
  n213 = Subtract(x=w153, y=w156) -> (x-y=w155:dbl)
  n214 = Add Array Elements(numeric array=w175) -> (sum=→"TP (<=0.4Hz)  2":dbl)
  n215 = Array Subset(array=w47, length=w50) -> (w38:dbl[])  [unwired: 1 in]
  n216 = Subtract(x=w218, y=w221) -> (x-y=w220:dbl)
  n217 = Add Array Elements(numeric array=w240) -> (sum=→"TP (<=0.4Hz)  2":dbl)
  n218 = Divide(x=0.04, y=w277) -> (x/y=w286:dbl)
  n219 = Array Subset(array=w98, index=w88, length=w89) -> (w86:dbl[])
  n220 = Subtract(x=w283, y=w286) -> (x-y=w285:dbl)
  n221 = Array Subset(array=w163, index=w153, length=w154) -> (w151:dbl[])
  n222 = Array Subset(array=w98, index=w91, length=w90) -> (w87:dbl[])
  n223 = Add Array Elements(numeric array=w305) -> (sum=→"TP (<=0.4Hz)":dbl)
  n224 = Array Subset(array=w228, index=w218, length=w219) -> (w216:dbl[])
  n225 = Array Subset(array=w163, index=w156, length=w155) -> (w152:dbl[])
  n226 = Array Subset(array=w228, index=w221, length=w220) -> (w217:dbl[])
  n227 = Array Subset(array=w293, index=w283, length=w284) -> (w281:dbl[])
  n228 = Absolute Value(x=w38) -> (abs(x)=w37:dbl[])
  n229 = Array Subset(array=w293, index=w286, length=w285) -> (w282:dbl[])
  n230 = Add Array Elements(numeric array=w87) -> (sum=w107:dbl)
  "LF  2" <- w107
  n231 = Add Array Elements(numeric array=w86) -> (sum=w106:dbl)
  "HF  2" <- w106
  n232 = Square(x=w37) -> (x^2=w36:dbl[])
  n233 = Add Array Elements(numeric array=w152) -> (sum=w172:dbl)
  "LF  2" <- w172
  n234 = Add Array Elements(numeric array=w151) -> (sum=w171:dbl)
  "HF  2" <- w171
  n235 = Add Array Elements(numeric array=w217) -> (sum=w237:dbl)
  "LF  2" <- w237
  n236 = Add Array Elements(numeric array=w216) -> (sum=w236:dbl)
  "HF  2" <- w236
  n237 = Add Array Elements(numeric array=w282) -> (sum=w302:dbl)
  "LF" <- w302
  n238 = Add Array Elements(numeric array=w281) -> (sum=w301:dbl)
  "HF" <- w301
  n239 = Divide(x=1.0, y=w33) -> (x/y=w35:dbl)
  n240 = Divide(x=w107, y=w106) -> (x/y=→"LF/HF 4":dbl)
  n241 = Divide(x=w172, y=w171) -> (x/y=→"LF/HF 3":dbl)
  n242 = Divide(x=w237, y=w236) -> (x/y=→"LF/HF 2":dbl)
  n243 = Multiply(x=w36, y=w35) -> (x*y=w34:dbl[])
  n244 = Divide(x=w302, y=w301) -> (x/y=→"LF/HF":dbl)
  n245 = Divide(x=1.0, y=w33) -> (x/y=w39:dbl)
  n246 = Array Size(array=w34) -> (size(s)=w31:i32)
  "psd_size 5" <- w31
  n247 = Bundle("x"=0.0, w39, w34) -> (→"PS_WD_stimuli4" →"PS_WD_stimuli4":cluster{"x":dbl, dbl, dbl[]})  [unwired: 1 in]
  n248 = To Double Precision Float(number=w31) -> (double precision float=w20:dbl)
  n249 = Divide(x=0.5, y=w20) -> (x/y=w18:dbl)
  n250 = Divide(x=0.15, y=w18) -> (x/y=w24:dbl)
  n251 = Divide(x=0.4, y=w18) -> (x/y=w21:dbl)
  n252 = Array Subset(array=w34, index=0, length=w21) -> (w46:dbl[])
  n253 = Subtract(x=w21, y=w24) -> (x-y=w25:dbl)
  n254 = Divide(x=0.04, y=w18) -> (x/y=w27:dbl)
  n255 = Subtract(x=w24, y=w27) -> (x-y=w26:dbl)
  n256 = Add Array Elements(numeric array=w46) -> (sum=→"TP (<=0.4Hz)  2":dbl)
  n257 = Array Subset(array=w34, index=w24, length=w25) -> (w22:dbl[])
  n258 = Array Subset(array=w34, index=w27, length=w26) -> (w23:dbl[])
  n259 = Add Array Elements(numeric array=w23) -> (sum=w43:dbl)
  "LF  2" <- w43
  n260 = Add Array Elements(numeric array=w22) -> (sum=w42:dbl)
  "HF  2" <- w42
  n261 = Divide(x=w43, y=w42) -> (x/y=→"LF/HF 5":dbl)
